vi "Load Image.vi"(11 "Path to PNG file":path) -> (3 "Image Array":i32[](array[numeric]))   [LabVIEW 2018]
doc: "Loads a png image, and converts it to a binary (black / white).\n\nIf the image fails to load, a 320 x 168 element array is returned."
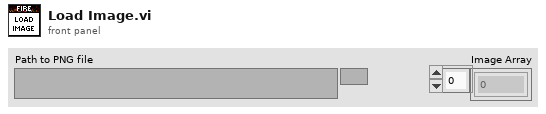
[diagram p1: front panel]
types:
  T1 = typedef "imagedata.ctl" = cluster{"image type":i32, "image depth":i32, "image":u8[], "mask":u8[], "colors":u32[], "Rectangle":cluster{"left":i16, "top":i16, "right":i16, "bottom":i16}}
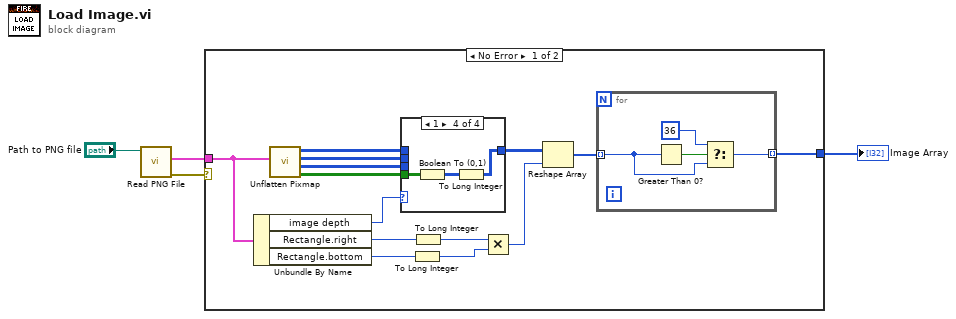
[diagram p0: block diagram]
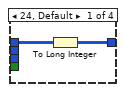
[diagram p2: hidden frame]
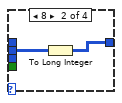
[diagram p3: hidden frame]
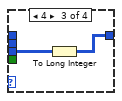
[diagram p4: hidden frame]
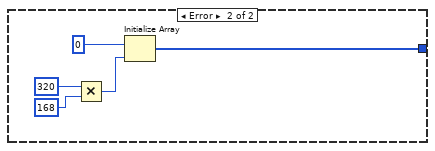
[diagram p5: hidden frame]
diagram:
  n1 = call <vilib>:"Read PNG File.vi"("path to PNG file"="Path to PNG file") -> ("error out"=w1:errorcluster, "image data"=w4:T1)  [unwired: 8 in, 1 out]
  n2 = case shown="No Error" w1 {
    tunnel: w4 -> [w18 _]
    tunnel: [w5 w35] -> w2
    frame No Error {
      n3 = Unbundle By Name(w18) -> ("image depth"=w11:i32, "Rectangle.right"=w17:i16, "Rectangle.bottom"=w16:i16)
      n4 = call <vilib>:"Unflatten Pixmap.vi"("image data"=w18) -> ("1-bit pixmap"=w6:bool[][], "4-bit pixmap"=w10:u8[][], "8-bit pixmap"=w9:u8[][], "24-bit pixmap"=w8:u32[][])  [unwired: 4 in, 3 out]
      n5 = case shown="1" w11 {
        tunnel: w10 -> [_ _ w24 _]
        tunnel: w9 -> [_ w21 _ _]
        tunnel: w8 -> [w19 _ _ _]
        tunnel: [w20 w22 w23 w25] -> w7
        tunnel: w6 -> [_ _ _ w27]
        frame 24, Default {
          n6 = To Long Integer(number=w19) -> (32bit integer=w20:i32[][])
        }
        frame 8 {
          n7 = To Long Integer(number=w21) -> (32bit integer=w22:i32[][])
        }
        frame 4 {
          n8 = To Long Integer(number=w24) -> (32bit integer=w23:i32[][])
        }
        frame 1 {
          n9 = Boolean To (0,1)(Boolean=w27) -> (0, 1=w26:i16[][])
          n10 = To Long Integer(number=w26) -> (32bit integer=w25:i32[][])
        }
      }
      n11 = To Long Integer(number=w16) -> (32bit integer=w13:i32)
      n12 = To Long Integer(number=w17) -> (32bit integer=w14:i32)
      n13 = Multiply(x=w14, y=w13) -> (x*y=w15:i32)
      n14 = Reshape Array(w7, w15) -> (w12:i32[])
      n15 = for {
        tunnel: w12 -> [w30] mode=indexing
        tunnel: [w28] -> w5 mode=indexing
        n16 = Greater Than 0?(x=w30) -> (x > 0?=w31:bool)
        n17 = Select(t=36, s=w31, f=w30) -> (s? t:f=w28:i32)
      }
    }
    frame Error {
      n18 = Multiply(x=320, y=168) -> (x*y=w32:i32)
      n19 = Initialize Array(0, w32) -> (w35:i32[])
    }
  }
  "Image Array" <- w2
